vi "0x2 RIO-OCU test.vi"() -> ()   [LabVIEW 2011]
uses:
  2-Think/2 Globals/2 Global.vi
  0x2 Classes/NetworkStreams/Writer/NetworkStreamWriter.lvclass
panel:
  out "Network \nfreq.":dbl
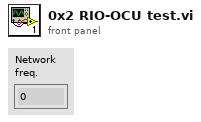
[diagram p1: front panel]
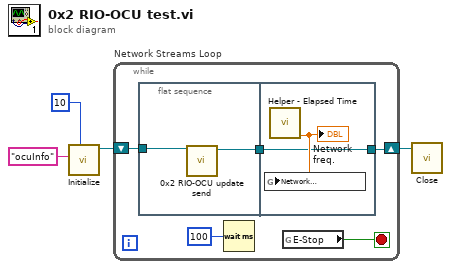
[diagram p0: block diagram]
diagram:
  n1 = call "Initialize.vi"("writer buffer size"=10, "writer name"="ocuInfo") -> ("NetworkStreamWriter out"=w2:refnum<class "NetworkStreamWriter.lvclass">)  [unwired: 8 in, 1 out]
  n2 = while "Network Streams Loop" {
    shift-right: [w6] -> w1
    shift-left: w2 -> [w7]
    stop <- w9 stop-if-true
    n3 = flat-sequence {
      tunnel: w7 -> [w11]
      tunnel: [w10] -> w5
      tunnel: [w12] -> w6
      tunnel: w5 -> [w12]
      frame #0 {
        n4 = call "0x2 RIO-OCU update send.vi"("OCU Writer In"=w11) -> ("OCU Writer Out"=w10:refnum<class "NetworkStreamWriter.lvclass">)  [unwired: 9 in, 1 out]
      }
      frame #1 {
        n5 = call "Helper - Elapsed Time.vi"() -> ("Frequency (Hz)"=w13:dbl)  [unwired: 10 in, 1 out]
        "Network \nfreq." <- w13
        n6 = global write "2 Global.vi" "Network \nfreq."(w13) -> ()
      }
    }
    n7 = Wait (ms)(milliseconds to wait=u32 100 ("millisecond multiple")) -> ()  [unwired: 1 out]
    n8 = global read "2 Global.vi" "E-Stop"() -> (w9:bool)
  }
  n9 = call "Close.vi"("NetworkStreamWriter in"=w1) -> ()  [unwired: 9 in, 2 out]
